vi "test_MyDLL.vi"() -> ()   [LabVIEW 2018]
uses:
  Cpp MyDll/MyDLL/MyDLL.dll
panel:
  out "vol":dbl
  out "sa 2":dbl
  in  "radius":dbl
  out "return type":i32
  out "error out":errorcluster
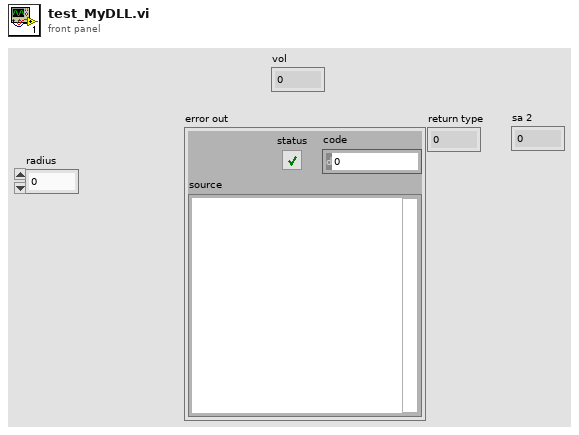
[diagram p1: front panel]
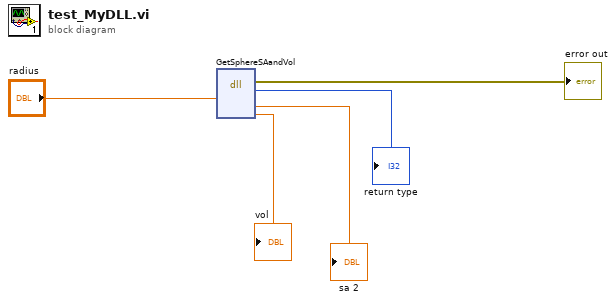
[diagram p0: block diagram]
diagram:
  n1 = dll-call lib="D:/codes labview/project dll-Cpp/Cpp MyDll/MyDLL/MyDLL.dll" fn="GetSphereSAandVol"("radius"="radius") -> (error out=→"error out":errorcluster, "return type"=→"return type":i32, "sa"=→"sa 2":dbl, "vol"=→"vol":dbl)  [unwired: 6 in, 1 out]
